vi "声发射_事件数.vi"(8 "波峰个数":i32, 9 "阈值":dbl format="%#_13g", 10 "位置":dbl[](array[numeric]), 11 "数据":dbl[](array[numeric])) -> (3 "事件数组":T1(array[cluster]))   [LabVIEW 2014]
panel:
  out "能量":dbl format="%#_13g"
  out "数值":i32
  out "波形图":dbl[](graph)
  out "结束位置":i32
  out "起始位置":i32
  out "事件数":i32
  out "flag":i32=-1
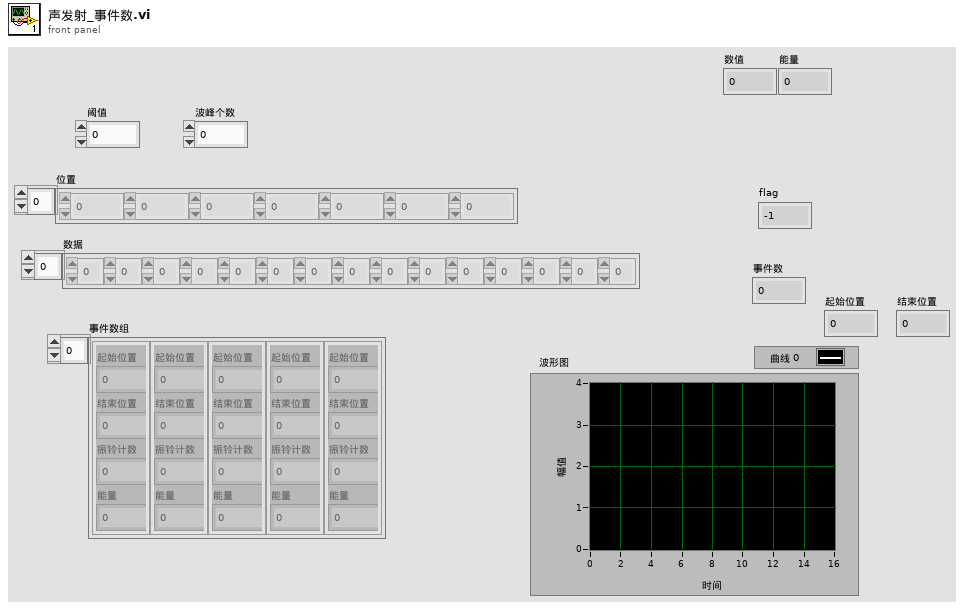
[diagram p1: front panel]
types:
  T1 = cluster{"起始位置":i32, "结束位置":i32, "振铃计数":i32, "能量":i32}[]
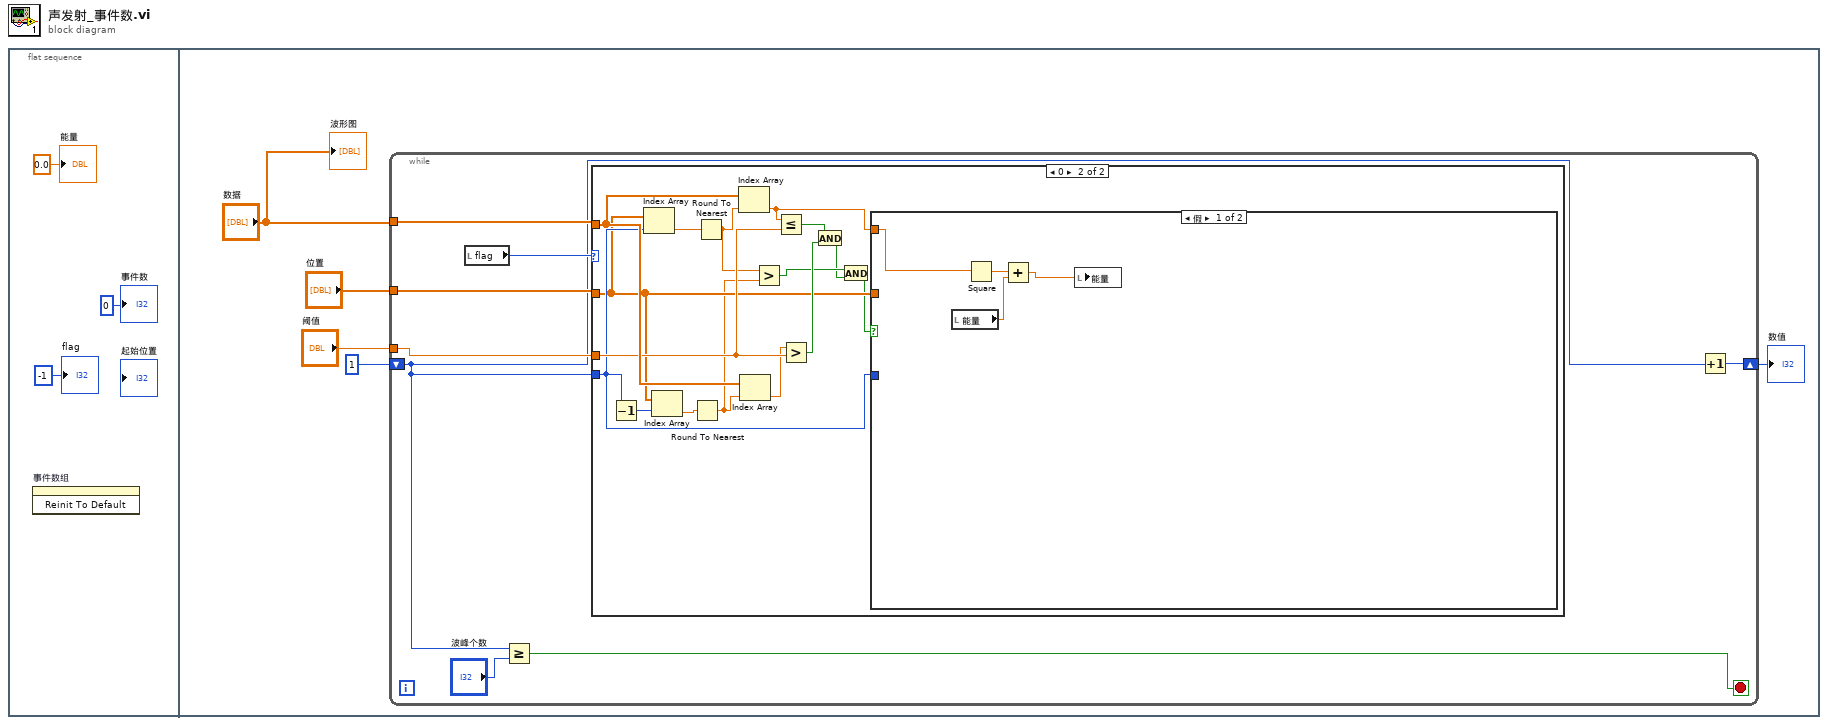
[diagram p0: block diagram]
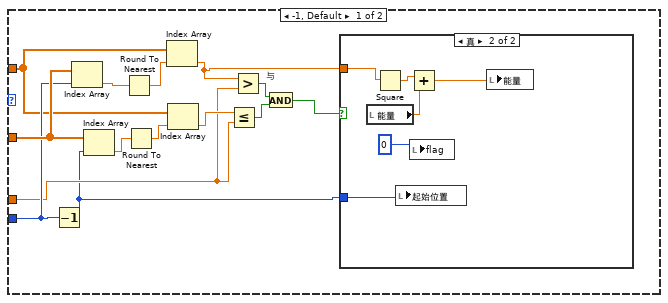
[diagram p2: hidden frame]
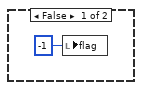
[diagram p3: hidden frame]
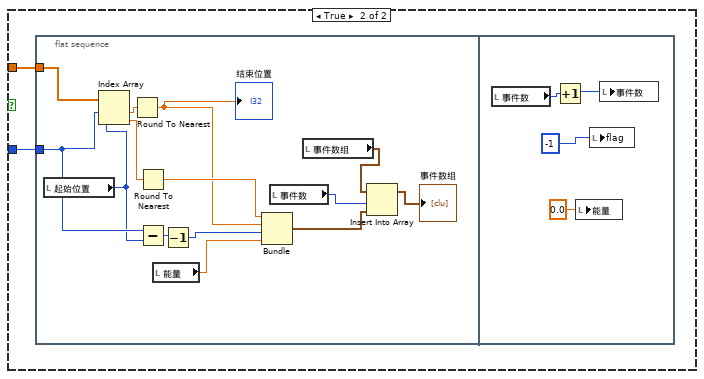
[diagram p4: hidden frame]
diagram:
  n1 = flat-sequence {
    frame #0 {
      n2 = invoke on="事件数组" class="Arr (严格)" method="Reinit To Default"() -> ()  [unwired: 3 in, 3 out]
      "事件数" <- 0 ("事件数")
      "flag" <- -1 ("数值")
      "能量" <- 0.0 ("能量")
    }
    frame #1 {
      n3 = while {
        tunnel: "位置" -> [w15]
        tunnel: "数据" -> [w14]
        shift-right: [w16] -> w4
        shift-left: 1 -> [w11]
        tunnel: "阈值" -> [w13]
        stop <- w9 stop-if-true
        n4 = local read "flag"() -> (w12:i32)
        n5 = Greater Or Equal?(x=w11, y="波峰个数") -> (x >= y?=w9:bool)
        n6 = case shown="0" w12 {
          tunnel: w15 -> [w28 w45]
          tunnel: w11 -> [w27 w46]
          tunnel: w14 -> [w24 w50]
          tunnel: w13 -> [w22 w49]
          frame -1, Default {
            n7 = Decrement(x=w27) -> (x-1=w18:i32)
            n8 = Index Array(array=w28, index=w27) -> (element=w30:dbl)
            n9 = Index Array(array=w28, index=w18) -> (element=w26:dbl)
            n10 = Round To Nearest(number=w30) -> (nearest integer value=w29:dbl)
            n11 = Round To Nearest(number=w26) -> (nearest integer value=w25:dbl)
            n12 = Index Array(array=w24, index=w29) -> (element=w17:dbl)
            n13 = Index Array(array=w24, index=w25) -> (element=w23:dbl)
            n14 = Less Or Equal?(x=w23, y=w22) -> (x <= y?=w20:bool)
            n15 = Greater?(x=w17, y=w22) -> (0:w21:bool)
            n16 = And "与"(x=w21, y=w20) -> (x .and. y?=w19:bool)
            n17 = case shown="真" w19 {
              tunnel: w18 -> [_ w36]
              tunnel: w17 -> [_ w35]
              frame False {
                n18 = local write "flag"(-1 ("数值")) -> ()
              }
              frame True {
                n19 = local read "能量"() -> (w33:dbl)
                n20 = Square(x=w35) -> (x^2=w34:dbl)
                n21 = local write "起始位置"(w36) -> ()
                n22 = Add(x=w34, y=w33) -> (x+y=w32:dbl)
                n23 = local write "flag"(0 ("数值 2")) -> ()
                n24 = local write "能量"(w32) -> ()
              }
            }
          }
          frame 0 {
            n25 = Decrement(x=w46) -> (x-1=w52:i32)
            n26 = Index Array(array=w45, index=w46) -> (element=w53:dbl)
            n27 = Index Array(array=w45, index=w52) -> (element=w51:dbl)
            n28 = Round To Nearest(number=w51) -> (nearest integer value=w43:dbl)
            n29 = Round To Nearest(number=w53) -> (nearest integer value=w44:dbl)
            n30 = Index Array(array=w50, index=w44) -> (element=w38:dbl)
            n31 = Index Array(array=w50, index=w43) -> (element=w39:dbl)
            n32 = Greater?(x=w44, y=w43) -> (0:w42:bool)
            n33 = Less Or Equal?(x=w38, y=w49) -> (x <= y?=w48:bool)
            n34 = Greater?(x=w39, y=w49) -> (0:w47:bool)
            n35 = And(x=w48, y=w47) -> (x .and. y?=w40:bool)
            n36 = And(x=w42, y=w40) -> (x .and. y?=w41:bool)
            n37 = case shown="假" w41 {
              tunnel: w46 -> [_ w59]
              tunnel: w45 -> [_ w58]
              tunnel: w38 -> [w57 _]
              frame False {
                n38 = local read "能量"() -> (w56:dbl)
                n39 = Square(x=w57) -> (x^2=w55:dbl)
                n40 = Add(x=w55, y=w56) -> (x+y=w54:dbl)
                n41 = local write "能量"(w54) -> ()
              }
              frame True {
                n42 = flat-sequence {
                  tunnel: w59 -> [w70]
                  tunnel: w58 -> [w69]
                  frame #0 {
                    n43 = local read "起始位置"() -> (w67:i32)
                    n44 = Index Array(array=w69, index #1=w70, index #2=w67) -> (element #1=w68:dbl, element #2=w66:dbl)
                    n45 = Round To Nearest(number=w68) -> (nearest integer value=w63:dbl)
                    "结束位置" <- w63
                    n46 = Round To Nearest(number=w66) -> (nearest integer value=w64:dbl)
                    n47 = Subtract(x=w70, y=w67) -> (x-y=w62:i32)
                    n48 = local read "能量"() -> (w60:dbl)
                    n49 = Decrement(x=w62) -> (x-1=w61:i32)
                    n50 = Bundle(w64, w63, w61, "能量"=w60) -> (w65:cluster{dbl, dbl, i32, "能量":dbl})  [unwired: 1 in]
                    n51 = local read "事件数"() -> (w71:i32)
                    n52 = local read "事件数组"() -> (w72:T1)
                    n53 = Insert Into Array(array=w72, index=w71, new element=w65) -> (→"事件数组":T1)
                  }
                  frame #1 {
                    n54 = local read "事件数"() -> (w75:i32)
                    n55 = Increment(x=w75) -> (x+1=w76:i32)
                    n56 = local write "能量"(0.0 ("能量")) -> ()
                    n57 = local write "flag"(-1 ("数值 2")) -> ()
                    n58 = local write "事件数"(w76) -> ()
                  }
                }
              }
            }
          }
        }
        n59 = Increment(x=w11) -> (x+1=w16:i32)
      }
      "数值" <- w4
      "波形图" <- "数据"
    }
  }
